vi "Write Document Name.vi"(8 "error in (no error)":errorcluster, 10 "Document Name":string, 11 "MDI serialize in":refnum<class "MDI serialize.lvclass">) -> (0 "error out":errorcluster, 3 "MDI serialize out":refnum<class "MDI serialize.lvclass">)   [LabVIEW 2019, in "MDI serialize.lvclass"]
uses:
  MDI serialize.lvclass
  MDI serialize.lvclass/MDI serialize.ctl
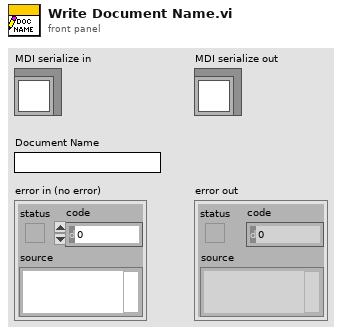
[diagram p1: front panel]
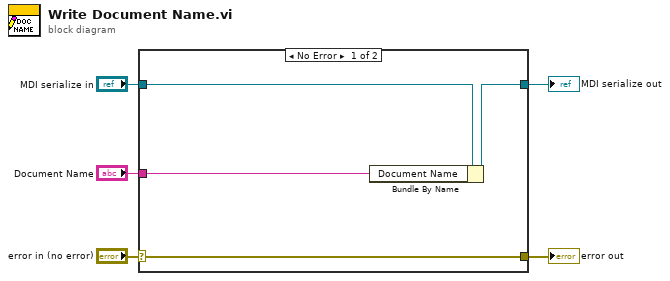
[diagram p0: block diagram]
diagram:
  n1 = case shown="No Error" "error in (no error)" {
    selector: "error in (no error)" -> [w9 w10]
    tunnel: [w9 w10] -> w4
    tunnel: [w7 w11] -> w2
    tunnel: "MDI serialize in" -> [w8 w11]
    tunnel: "Document Name" -> [w6 _]
    frame No Error {
      n2 = Bundle By Name(cluster=w8, "Document Name"=w6) -> (w7:refnum<class "MDI serialize.lvclass">)
    }
    frame Error {
    }
  }
  "error out" <- w4
  "MDI serialize out" <- w2
